vi "addVoxelsToLines.vi"(8 "error in":errorcluster, 10 "Queues":T2, 11 "FPGA VI ref":T1) -> (0 "error out":errorcluster, 2 "num elements available":u32, 4 "num elements requested":u32, 5 "lines with no data":i32, 6 "num read":u32, 7 "lines read":u32)   [LabVIEW 2010]
uses:
  internal_queues.ctl
  line_info.ctl
  volume_with_lines.ctl
  volume_info.ctl
  FPGA_ref.ctl
  <vilib>/rvi/interface/nirviMethod/nirviMethod.xnode
  <vilib>/rvi/interface/common/niFpgaNodeNameForErrorReporting.ctl
  <vilib>/rvi/errors/niLvFpgaWhatHappensToTopLevelVI.ctl
  <vilib>/rvi/interface/nirviReadWriteControl/nirviReadWriteControl.xnode
  <vilib>/Utility/error.llb/Error Cluster From Error Code.vi
  <vilib>/rvi/errors/niLvFpgaAdjustHostInterfaceError.vi
  NiFpgaLv.dll
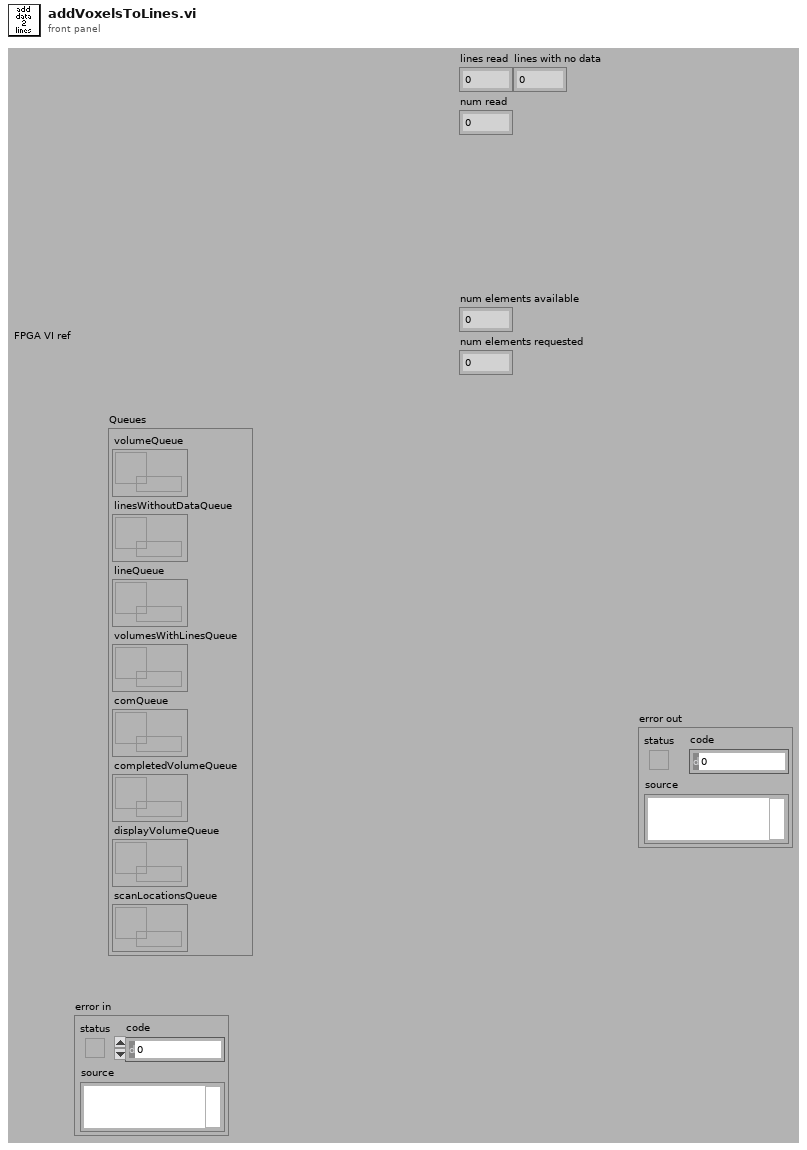
[diagram p1: front panel]
types:
  T1 = typedef "FPGA_ref.ctl" = refnum<k20>
  T2 = typedef "internal_queues.ctl" = cluster{"volumeQueue":refnum<queue>, "linesWithoutDataQueue":refnum<queue>, "lineQueue":refnum<queue>, "volumesWithLinesQueue":refnum<queue>, "comQueue":refnum<queue>, "completedVolumeQueue":refnum<queue>, "displayVolumeQueue":refnum<queue>, "scanLocationsQueue":refnum<queue>}
  T3 = typedef "niFpgaNodeNameForErrorReporting.ctl" = enum16{"Open FPGA VI Reference", "Read/Write Control", "Invoke Method: Abort", "Invoke Method: Acknowledge IRQ", "Invoke Method: Download", "Invoke Method: FIFO.Configure", "Invoke Method: FIFO.Read", "Invoke Method: FIFO.Start", "Invoke Method: FIFO.Stop", "Invoke Method: FIFO.Write", "Invoke Method: Reset", "Invoke Method: Run", "Invoke Method: Wait on IRQ", "Close FPGA VI Reference"}
  T4 = typedef "niLvFpgaWhatHappensToTopLevelVI.ctl" = enum16{"top level VI scripted behind XNode", "top level VI inlined behind XNode"}
  T5 = typedef "line_info.ctl" = cluster{"start X":i16, "start Y":i16, "start Z":i16, "end X":i16, "end Y":i16, "end Z":i16, "num z":u8, "voxel data":u32[], "volume num":u32, "line number":u16, "frame number":u16}
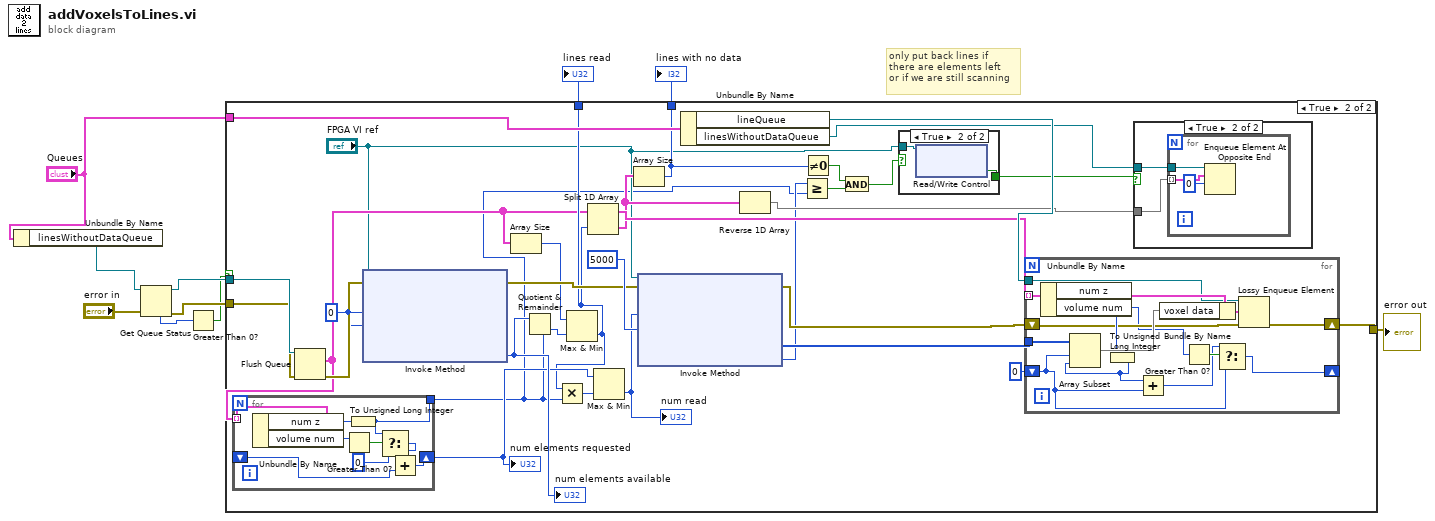
[diagram p0: block diagram]
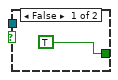
[diagram p3: hidden frame]
diagram:
  # "only put back lines if\nthere are elements left\nor if we are still scanning"
  n1 = Unbundle By Name("Queues") -> ("linesWithoutDataQueue"=w9:refnum<queue>)
  n2 = Get Queue Status(queue=w9, error in (no error)="error in") -> (queue out=w7:refnum<queue>, error out=w6:errorcluster, # elements in queue=w8:i32)  [unwired: 1 in, 5 out]
  n3 = Greater Than 0?(x=w8) -> (x > 0?=w4:bool)
  n4 = case shown="True" w4 {
    tunnel: "Queues" -> [_ w25]
    tunnel: w7 -> [_ w40]
    tunnel: w6 -> [w11 w39]
    tunnel: [w11 w38] -> w3
    tunnel: [_ w23] -> w2
    tunnel: [_ w19] -> w1
    frame False {
    }
    frame True {
      w36 = u32 0 ("Number of Elements")
      n5 = Flush Queue(queue=w40, error in (no error)=w39) -> (remaining elements=w22:T5[], error out=w37:errorcluster)  [unwired: 1 out]
      n6 = for {
        tunnel: w22 -> [w103] mode=indexing
        shift-right: [w102] -> w24
        shift-left: _ -> [w96]
        tunnel: [w95] -> w12
        n7 = Unbundle By Name(w103) -> ("num z"=w99:u8, "volume num"=w101:u32)
        n8 = Greater Than 0?(x=w101) -> (x > 0?=w100:bool)
        n9 = To Unsigned Long Integer(number=w99) -> (unsigned 32bit integer=w95:u32)
        n10 = Select(t=w95, s=w100, f=u32 0) -> (s? t:f=w97:u32)
        n11 = Add(x=w97, y=w96) -> (x+y=w102:u32)
      }
      "num elements requested" <- w24
      n12 = xnode "Invoke Method"("FPGA VI Reference In"="FPGA VI ref", "error in"=w37, "Number of Elements"=w36, "Timeout (ms)"=w36) -> ("error out"=w29:errorcluster, "Elements Remaining"=w35:u32)  [unwired: 2 out]
      "num elements available" <- w35
      n13 = Array Size(array=w22) -> (size(s)=w21:i32)
      n14 = Quotient & Remainder(x=w35, y=w12) -> (floor(x/y)=w20:u32)  [unwired: 1 out]
      n15 = Max & Min(x=w21, y=w20) -> (min(x,y)=w23:u32)  [unwired: 1 out]
      n16 = Multiply(x=w23, y=w12) -> (x*y=w34:u32)
      n17 = Split 1D Array(array=w22, index=w23) -> (first subarray=w32:T5[], second subarray=w28:T5[])
      n18 = Max & Min(x=w24, y=w34) -> (min(x,y)=w33:u32)  [unwired: 1 out]
      "num read" <- w33
      n19 = Array Size(array=w28) -> (size(s)=w19:i32)
      n20 = xnode "Invoke Method"("FPGA VI Reference In"="FPGA VI ref", "error in"=w29, "Number of Elements"=w33, "Timeout (ms)"=5000) -> ("error out"=w26:errorcluster, "Data"=w27:u32[], "Elements Remaining"=w13:u32)  [unwired: 1 out]
      n21 = Unbundle By Name(w25) -> ("lineQueue"=w43:refnum<queue>, "linesWithoutDataQueue"=w30:refnum<queue>)
      n22 = Reverse 1D Array(array=w28) -> (reversed array=w31:T5[])
      n23 = Greater Or Equal?(x=w13, y=w12) -> (x >= y?=w18:bool)
      n24 = Not Equal To 0?(x=w19) -> (x != 0?=w17:bool)
      n25 = And(x=w17, y=w18) -> (x .and. y?=w15:bool)
      n26 = case shown="True" w15 {
        tunnel: "FPGA VI ref" -> [_ w46]
        tunnel: [TRUE ("scanning?") w45] -> w14
        frame False {
        }
        frame True {
          n27 = xnode "Read/Write Control"("FPGA VI Reference In"=w46) -> ("scanning?"=w45:bool)  [unwired: 1 in, 2 out]
        }
      }
      n28 = for {
        tunnel: w32 -> [w189] mode=indexing
        tunnel: w27 -> [w190]
        shift-right: [w178] -> _
        shift-left: u32 0 -> [w179]
        shift-right: [w183] -> w38
        shift-left: w26 -> [w184]
        tunnel: w43 -> [w185]
        n29 = Unbundle By Name(w189) -> ("num z"=w187:u8, "volume num"=w182:u32)
        n30 = To Unsigned Long Integer(number=w187) -> (unsigned 32bit integer=w177:u32)
        n31 = Array Subset(array=w190, index=w179, length=w177) -> (w188:u32[])
        n32 = Add(x=w177, y=w179) -> (x+y=w180:u32)
        n33 = Bundle By Name(cluster=w189, "voxel data"=w188) -> (w186:T5)
        n34 = Greater Than 0?(x=w182) -> (x > 0?=w181:bool)
        n35 = Select(t=w180, s=w181, f=w179) -> (s? t:f=w178:u32)
        n36 = Lossy Enqueue Element(queue=w185, element=w186, error in (no error)=w184) -> (error out=w183:errorcluster)  [unwired: 3 out]
      }
      n37 = case shown="True" w14 {
        tunnel: w31 -> [_ w91]
        tunnel: w30 -> [_ w90]
        frame False {
        }
        frame True {
          n38 = for {
            tunnel: w91 -> [w94] mode=indexing
            tunnel: w90 -> [w93]
            n39 = Enqueue Element At Opposite End(queue=w93, element=w94, timeout in ms (-1)=0) -> ()  [unwired: 1 in, 3 out]
          }
        }
      }
    }
  }
  "error out" <- w3
  "lines read" <- w2
  "lines with no data" <- w1
